vi "Main VI Template.vi"(8 "Error In":errorcluster, 11 "MainData":T1) -> (0 "Error Out":errorcluster, 3 "MainData out":T1)   [LabVIEW 2019, in "MainController.lvlib"]
uses:
  Cluster - MainData.ctl
  All Message Queues.ctl
  Cluster - MainControllerMessage.ctl
  Enum - MainState.ctl
  AutoMode/Cluster - AutoModeMessage.ctl
  AutoMode/Enum - AutoModeState.ctl
  ManualMode/Cluster - ManualModeMessageCluster.ctl
  ManualMode/Enum - ManualModeMessage.ctl
  Settings/CTL_MessageCluster.ctl
  Settings/CTL_SettingsMessage.ctl
  Cluster - HardwareConfiguration.ctl
  Cluster - LoggingConfiguration.ctl
  Cluster - TestSettings.ctl
  UI State.ctl
  UI Data.ctl
  MainController.lvlib
  AutoMode/AutoMode.lvlib
  ManualMode/ManualMode.lvlib
  Settings/Settings.lvlib
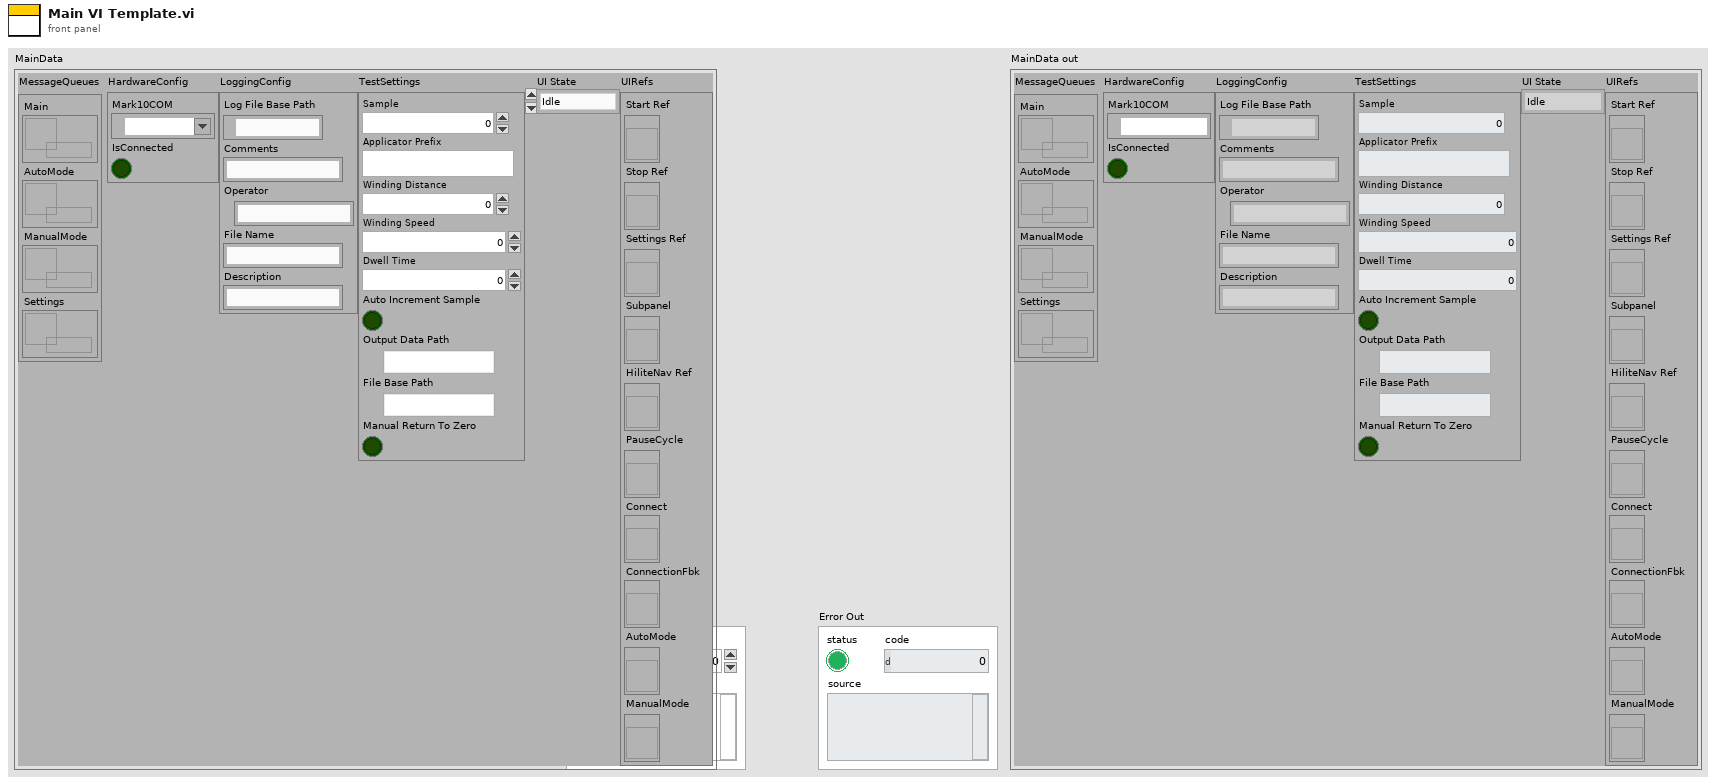
[diagram p1: front panel]
types:
  T1 = typedef "MainController.lvlib/Cluster - MainData.ctl" = cluster{"MessageQueues":T2, "HardwareConfig":T3, "LoggingConfig":T4, "TestSettings":T5, "UI State":T6, "UIRefs":T7}
  T2 = typedef "MainController.lvlib/All Message Queues.ctl" = cluster{"Main":refnum<queue>, "AutoMode":refnum<queue>, "ManualMode":refnum<queue>, "Settings":refnum<queue>}
  T3 = typedef "MainController.lvlib/Cluster - HardwareConfiguration.ctl" = cluster{"Mark10COM":refnum<visa-resource-name>, "IsConnected":bool}
  T4 = typedef "MainController.lvlib/Cluster - LoggingConfiguration.ctl" = cluster{"Log File Base Path":path, "Comments ":string, "Operator":string, "File Name":string, "Description":string}
  T5 = typedef "MainController.lvlib/Cluster - TestSettings.ctl" = cluster{"Sample":u32, "Applicator Prefix":string, "Winding Distance":dbl, "Winding Speed":dbl, "Dwell Time":dbl, "Auto Increment Sample":bool, "Output Data Path":path, "File Base Path":path, "Manual Return To Zero":bool}
  T6 = typedef "MainController.lvlib/UI State.ctl" = enum16{"Idle", "AutoIdle", "AutoRunning", "ManualMode", "Settings"}
  T7 = typedef "MainController.lvlib/UI Data.ctl" = cluster{"Start Ref":refnum<vi>, "Stop Ref":refnum<vi>, "Settings Ref":refnum<vi>, "Subpanel":refnum<vi>, "HiliteNav Ref":refnum<vi>, "PauseCycle":refnum<vi>, "Connect":refnum<vi>, "ConnectionFbk":refnum<vi>, "AutoMode":refnum<vi>, "ManualMode":refnum<vi>}
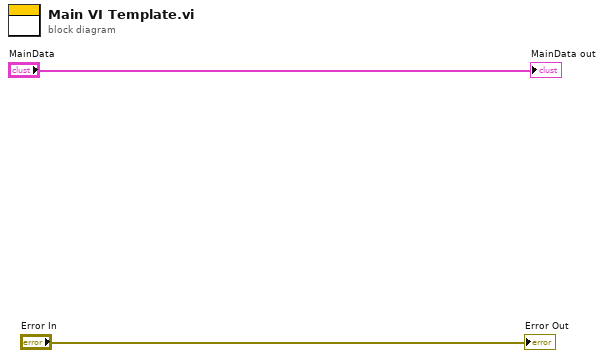
[diagram p0: block diagram]
diagram:
  "Error Out" <- "Error In"
  "MainData out" <- "MainData"
